vi "Configure Power Measurement List.vi"(6 "Exp Nominal Power":dbl[](array[numeric]) format="%^.3e", 7 "List Length (10)":i32=10, 8 "error in (no error)":errorcluster, 10 "Instance (1)":i32=1 format="%.0g", 11 "VISA resource name":refnum<visa-resource-name>) -> (0 "error out":errorcluster, 3 "VISA resource name out":refnum<visa-resource-name>)   [LabVIEW 2020, in "Rohde&Schwarz CMXP GPRF.lvlib"]
doc: "Configures list of power measurement points.\n\nAttribute:\nRSCMXPGPRF_ATTR_POWER_MEASUREMENT_EXPECTED_NOMINAL_POWER_ALL\n\nRemote-control command:\nCONFigure:GPRF:MEAS<i>:POWer:LIST:ENPower:ALL"
uses:
  <instrlib>/Rohde&Schwarz CMXP GPRF/Rohde&Schwarz CMXP GPRF.lvlib
  <instrlib>/Rohde&Schwarz CMXP GPRF/Private/rsidr_core.llb/rsidr_core.lvlib
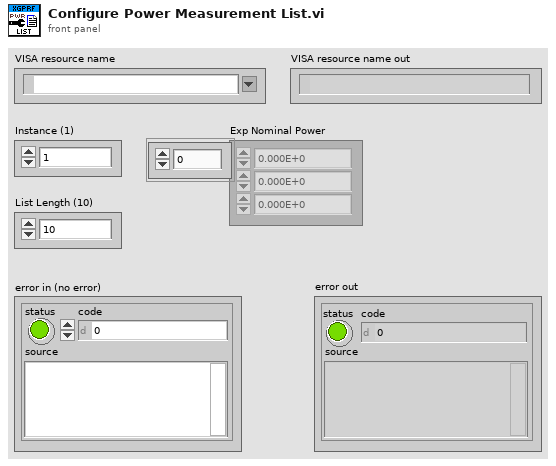
[diagram p1: front panel]
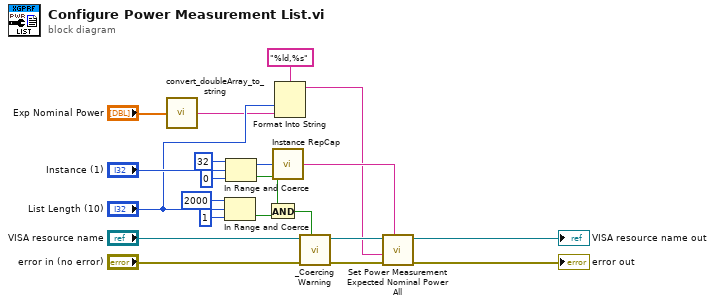
[diagram p0: block diagram]
diagram:
  n1 = call <instrlib>:"convert_doubleArray_to_string.vi"("double array in"="Exp Nominal Power") -> ("string out"=w2:string)  [unwired: 4 in]
  n2 = In Range and Coerce(upper limit=2000, x="List Length (10)", lower limit=1) -> (In Range?=w16:bool)  [unwired: 1 out]
  n3 = In Range and Coerce(upper limit=32, x="Instance (1)", lower limit=0) -> (coerced(x)=w6:i32, In Range?=w15:bool)
  n4 = And(x=w15, y=w16) -> (x .and. y?=w17:bool)
  n5 = call <instrlib>:"Instance RepCap.vi"("Instance in"=w6) -> ("Instance out"=w5:string)
  n6 = Format Into String(format string="%ld,%s", "List Length (10)", w2) -> (resulting string=w1:string)  [unwired: 2 in, 1 out]
  n7 = call <instrlib>:"_Coercing Warning.vi"("In Range?"=w17, "error in (no error)"="error in (no error)", "VISA resource name"="VISA resource name") -> ("error out"=w11:errorcluster, "VISA resource name out"=w10:refnum<visa-resource-name>)  [unwired: 7 in]
  n8 = call "Set Power Measurement Expected Nominal Power All"("Repeated Capabilities"=w5, "error in (no error)"=w11, "Power Measurement Expected Nominal Power All ()"=w1, "instrument handle"=w10) -> ("error out"=→"error out":errorcluster, "instrument handle out"=→"VISA resource name out":refnum<visa-resource-name>)  [unwired: 6 in]
